vi "test_StopSMO.vi"(8 "error in (no error)":errorcluster, 11 "TestCase in":refnum<class "SMO_TestCase.lvclass">) -> (0 "error out":errorcluster, 3 "TestCase out":refnum<class "SMO_TestCase.lvclass">)   [LabVIEW 2013, in "SMO_TestCase.lvclass"]
uses:
  SMO_TestCase.lvclass
  SMO_TestCase.lvclass/SMO_TestCase.ctl
  <vilib>/addons/_JKI Toolkits/VI Tester/TestCase.llb/TestCase.lvclass
  src/SMO/SMO.lvclass
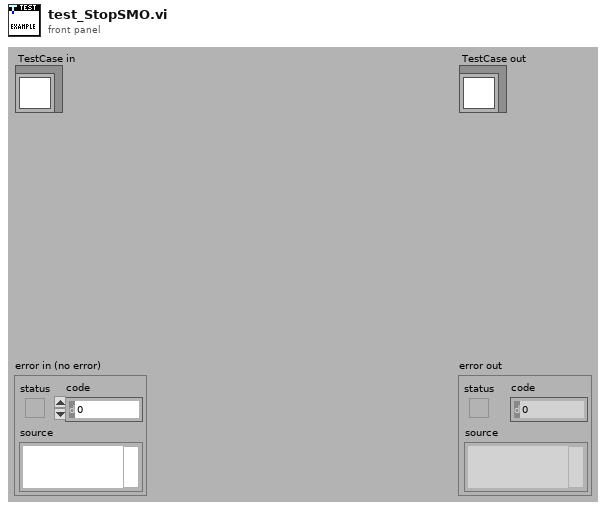
[diagram p1: front panel]
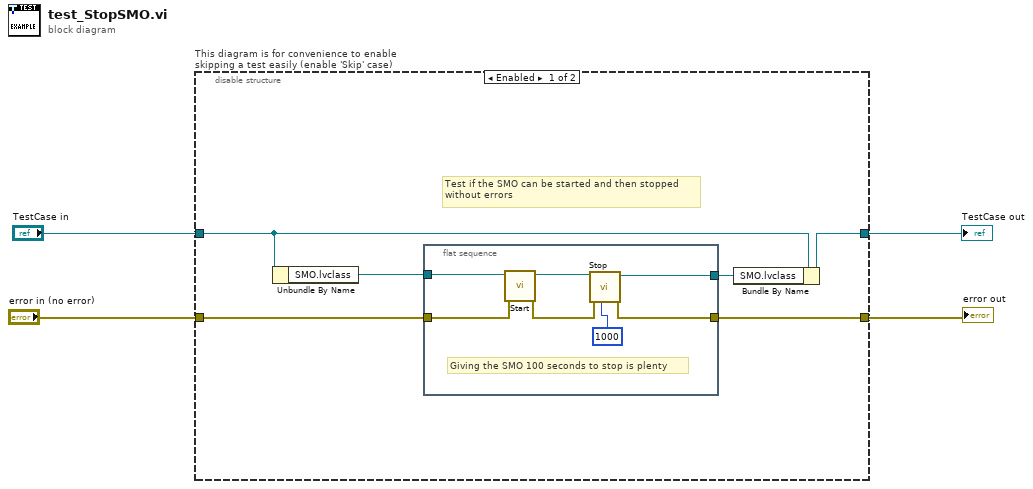
[diagram p0: block diagram]
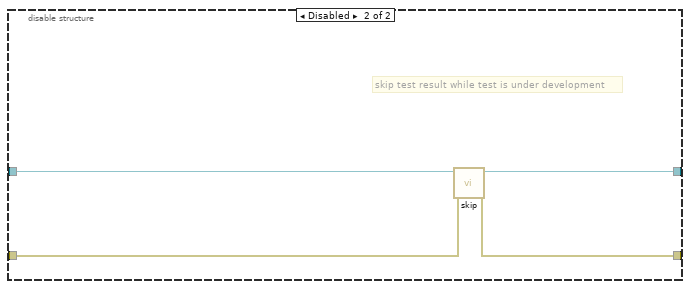
[diagram p2: hidden frame]
diagram:
  n1 = disable-structure "This diagram is for convenience to enable skipping a test easily (enable 'Skip' case)" shown="Enabled" {
    disable-tunnel: "TestCase in" -> [w6 w21]
    disable-tunnel: [w5 w19] -> w1
    disable-tunnel: [w8 w20] -> w3
    disable-tunnel: "error in (no error)" -> [w9 w18]
    frame Enabled {
      # "Test if the SMO can be started and then stopped\nwithout errors"
      n2 = Unbundle By Name(w6) -> ("SMO.lvclass"=w10:refnum<class "SMO.lvclass">)
      n3 = flat-sequence {
        tunnel: w10 -> [w17]
        tunnel: w9 -> [w16]
        tunnel: [w13] -> w8
        tunnel: [w11] -> w7
        frame #0 {
          # "Giving the SMO 100 seconds to stop is plenty"
          n4 = call "Start.vi"("error in (no error)"=w16, "SMO"=w17) -> ("error out"=w14:errorcluster, "SMO out"=w15:refnum<class "SMO.lvclass">)  [unwired: 8 in]
          n5 = call "Stop.vi"("timeout in ms (-1)"=1000, "error in (no error)"=w14, "SMO"=w15) -> ("error out"=w13:errorcluster, "SMO out"=w11:refnum<class "SMO.lvclass">)  [unwired: 7 in]
        }
      }
      n6 = Bundle By Name(cluster=w6, "SMO.lvclass"=w7) -> (w5:refnum<class "SMO_TestCase.lvclass">)
    }
    frame Disabled {
      # "skip test result while test is under development"
      n7 = call <vilib>:"skip.vi"("error in (no error)"=w18, "TestCase in"=w21) -> ("error out"=w20:errorcluster, "TestCase out"=w19:refnum<class "SMO_TestCase.lvclass">)  [unwired: 8 in]
    }
  }
  "error out" <- w3
  "TestCase out" <- w1
